vi "AB_RW_Project_RESTfulWebService_Info.vi"(7 "action":T5, 8 "error in (no error)":errorcluster, 10 "RESTfulWebServiceInfo in":T1, 11 "Object In":T6) -> (0 "error out":errorcluster, 2 "RESTfulWebServiceInfo out":T1, 3 "Object Out":T6)   [LabVIEW 2020]
uses:
  <resource>/Framework/Providers/API/ItemRef.ctl
  <vilib>/AppBuilder/RW_Project/AB_RW_Project_PropBag_Action.ctl
  <vilib>/AppBuilder/RW_Project/AB_RW_Project_RESTfulWebService_Data.ctl
  <vilib>/AppBuilder/RW_Project/AB_RW_Project_RESTful_RoutingTemplate.ctl
  <vilib>/AppBuilder/AB_Classes/RESTful/AB_RESTful_RoutingType.ctl
  <vilib>/AppBuilder/AB_Classes/RESTful/AB_RESTful_HTTPMethodType.ctl
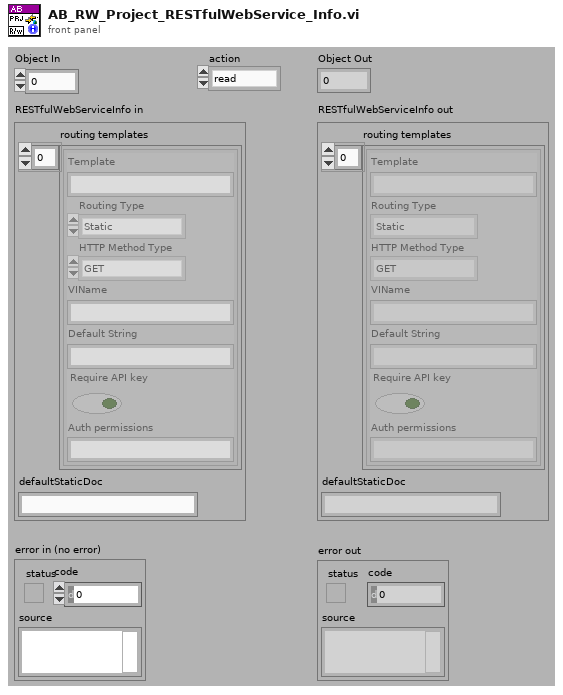
[diagram p1: front panel]
types:
  T1 = typedef "AB_RW_Project_RESTfulWebService_Data.ctl" = cluster{"routing templates":T2[], "defaultStaticDoc":string}
  T2 = typedef "AB_RW_Project_RESTful_RoutingTemplate.ctl" = cluster{"Template":string, "Routing Type":T3, "HTTP Method Type":T4, "VIName":string, "Default String":string, "Require API key":bool, "Auth permissions":string}
  T3 = typedef "AB_RESTful_RoutingType.ctl" = enum32{"Method", "Static"}
  T4 = typedef "AB_RESTful_HTTPMethodType.ctl" = enum32{"GET", "POST", "PUT", "DELETE"}
  T5 = typedef "AB_RW_Project_PropBag_Action.ctl" = enum16{"read", "write", "clear", "readPrevious", "writePrevious", "clearPrevious"}
  T6 = typedef "ItemRef.ctl" = u64
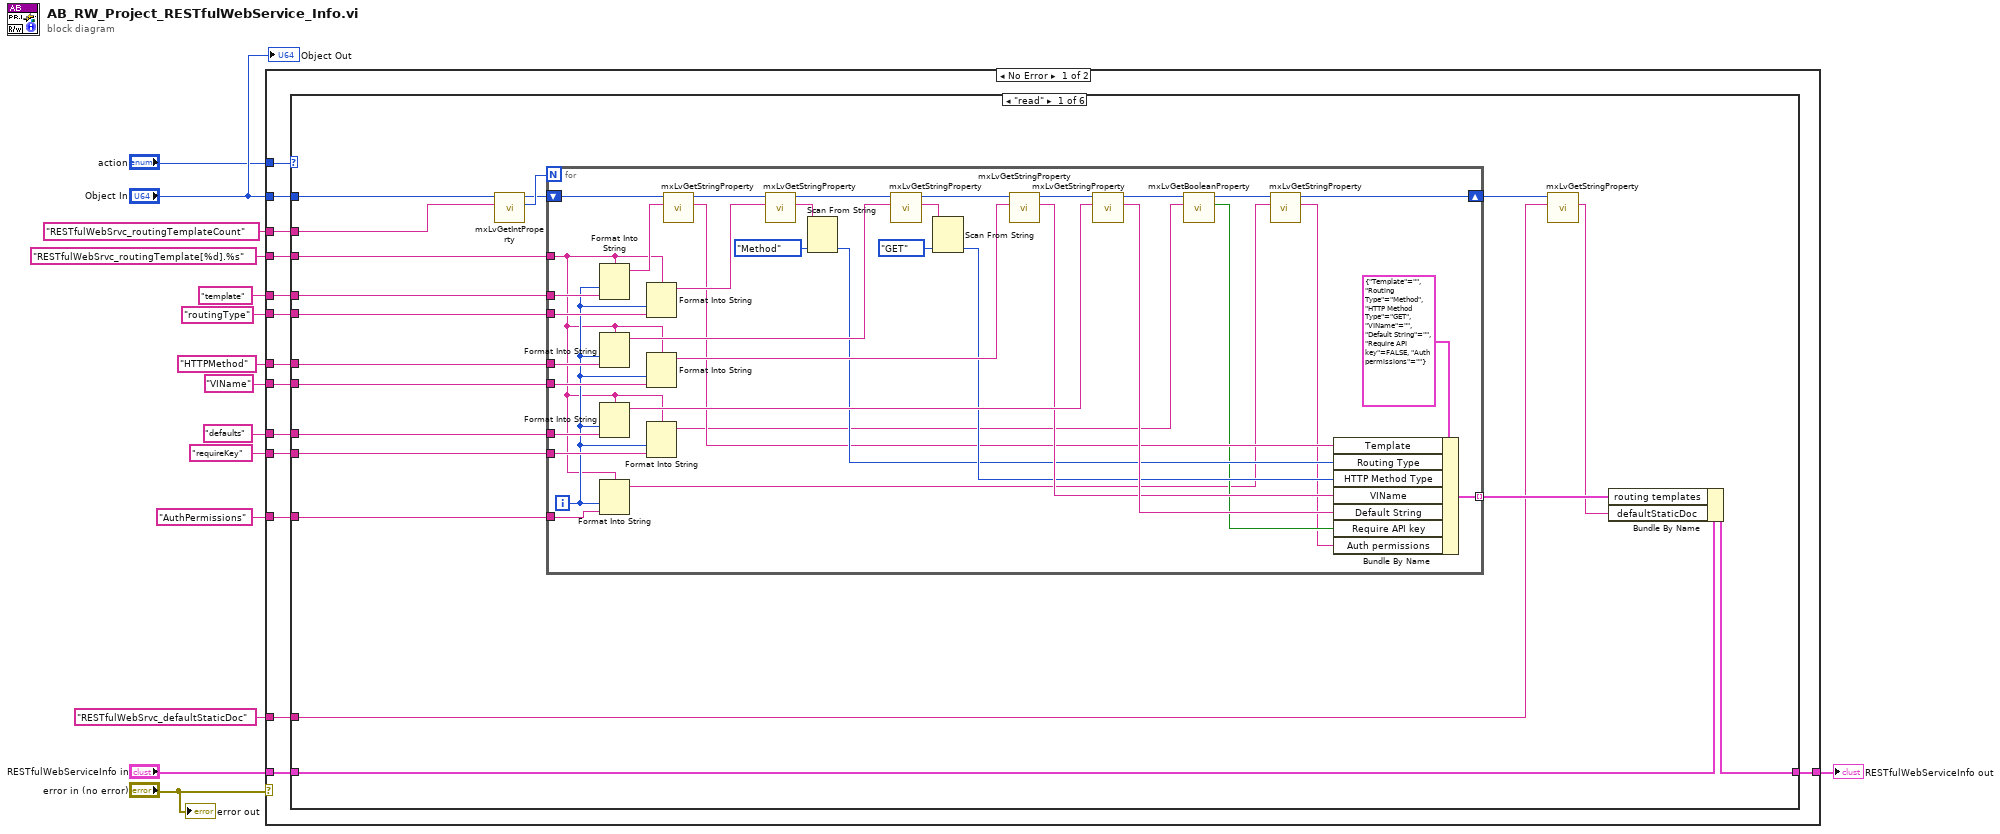
[diagram p0: block diagram]
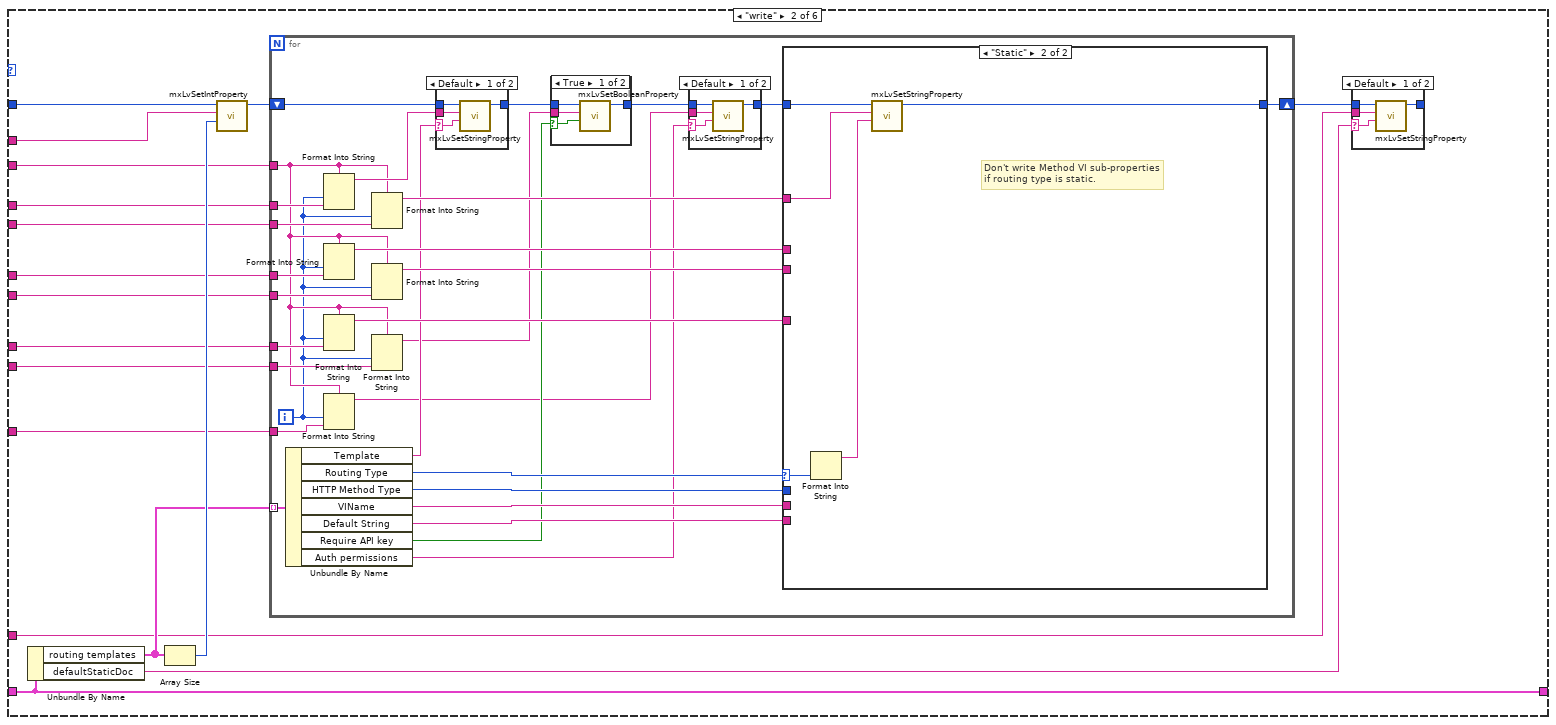
[diagram p2: hidden frame]
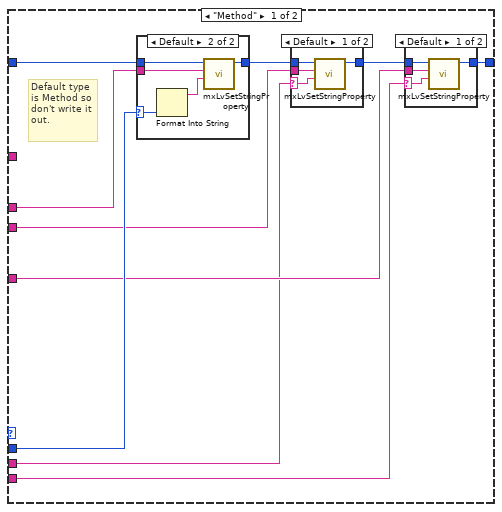
[diagram p6: hidden frame]
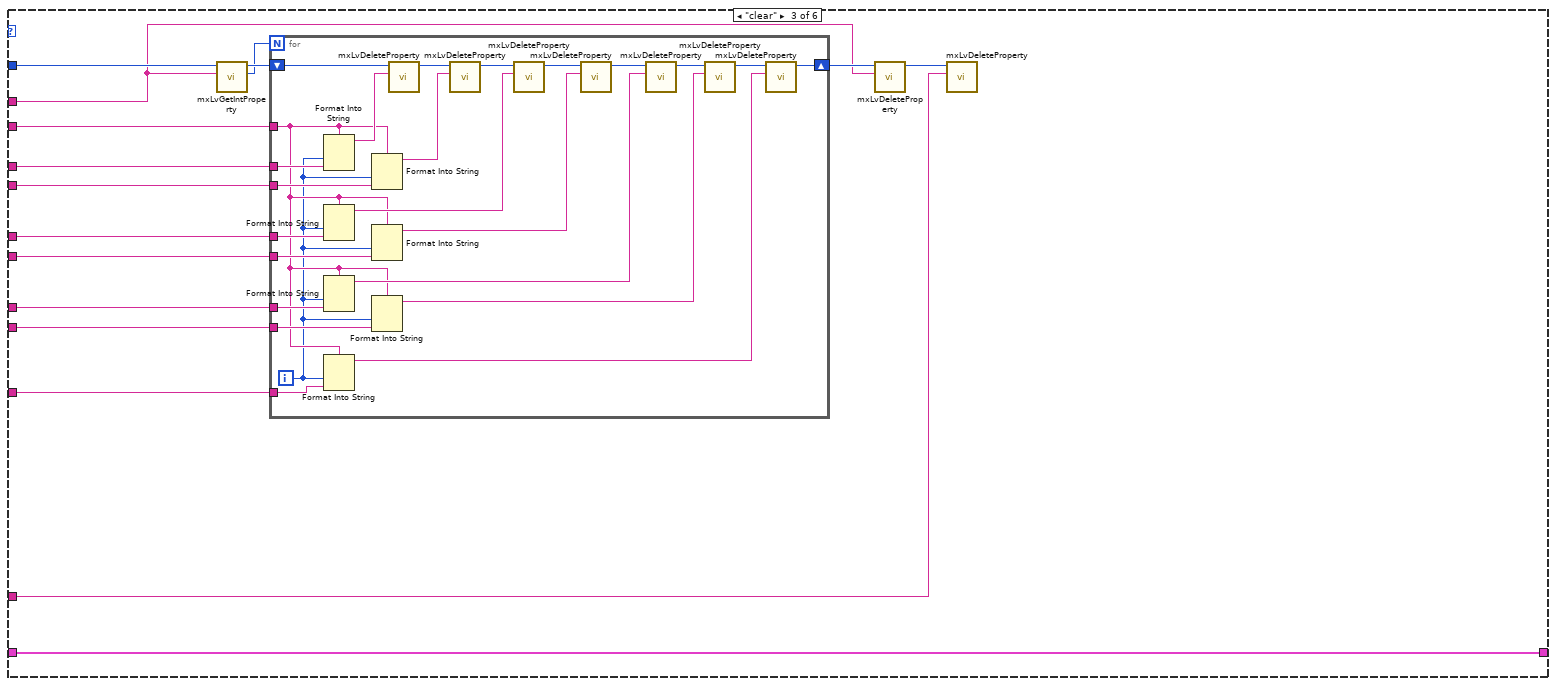
[diagram p11: hidden frame]
diagram:
  n1 = case shown="No Error" "error in (no error)" {
    tunnel: "Object In" -> [w29 _]
    tunnel: [w23 _] -> w8
    tunnel: "RESTfulWebSrvc_routingTemplateCount" ("Tag") -> [w28 _]
    tunnel: "RESTfulWebSrvc_routingTemplate[%d].%s" ("Tag") -> [w27 _]
    tunnel: "template" ("Tag") -> [w26 _]
    tunnel: "RESTfulWebServiceInfo in" -> [w25 _]
    tunnel: "action" -> [w24 _]
    tunnel: "routingType" ("Tag") -> [w22 _]
    tunnel: "HTTPMethod" ("Tag") -> [w21 _]
    tunnel: "VIName" ("Tag") -> [w20 _]
    tunnel: "defaults" ("Tag") -> [w19 _]
    tunnel: "requireKey" ("Tag") -> [w18 _]
    tunnel: "RESTfulWebSrvc_defaultStaticDoc" ("Tag") -> [w17 _]
    tunnel: "AuthPermissions" ("Tag") -> [w16 _]
    frame No Error {
      n2 = case shown="\"read\"" w24 {
        tunnel: w29 -> [w41 w98 w196 _ _ _]
        tunnel: w28 -> [w47 w100 w187 _ _ _]
        tunnel: w27 -> [w45 w96 w194 _ _ _]
        tunnel: w26 -> [w40 w95 w193 _ _ _]
        tunnel: w25 -> [w42 w99 w195 w222 w223 w224]
        tunnel: [w43 w99 w195 w222 w223 w224] -> w23
        tunnel: w22 -> [w39 w94 w192 _ _ _]
        tunnel: w21 -> [w38 w93 w191 _ _ _]
        tunnel: w20 -> [w37 w92 w190 _ _ _]
        tunnel: w19 -> [w36 w91 w189 _ _ _]
        tunnel: w18 -> [w34 w89 w186 _ _ _]
        tunnel: w17 -> [w32 w87 w183 _ _ _]
        tunnel: w16 -> [w30 w85 w182 _ _ _]
        frame "read" {
          n3 = call <resource>:"mxLvGetIntProperty.vi"("Tag"=w47, "Item"=w41) -> ("Value"=w46:i32, "Item"=w44:T6)  [unwired: 1 in, 7 out]
          n4 = for {
            N: w46 -> [_]
            shift-right: [w50] -> w33
            shift-left: w44 -> [w84]
            tunnel: w45 -> [w53]
            tunnel: w40 -> [w81]
            tunnel: w39 -> [w80]
            tunnel: w38 -> [w79]
            tunnel: w37 -> [w78]
            tunnel: w36 -> [w77]
            tunnel: [w60] -> w35 mode=indexing
            tunnel: w34 -> [w57]
            tunnel: w30 -> [w52]
            i -> [w54]
            n5 = Format Into String(format string=w53, w54, w81) -> (resulting string=w76:string)  [unwired: 2 in, 1 out]
            n6 = Format Into String(format string=w53, w54, w79) -> (resulting string=w71:string)  [unwired: 2 in, 1 out]
            n7 = Format Into String(format string=w53, w54, w77) -> (resulting string=w66:string)  [unwired: 2 in, 1 out]
            n8 = Format Into String(format string=w53, w54, w52) -> (resulting string=w48:string)  [unwired: 2 in, 1 out]
            n9 = Format Into String(format string=w53, w54, w80) -> (resulting string=w75:string)  [unwired: 2 in, 1 out]
            n10 = Format Into String(format string=w53, w54, w78) -> (resulting string=w67:string)  [unwired: 2 in, 1 out]
            n11 = Format Into String(format string=w53, w54, w57) -> (resulting string=w56:string)  [unwired: 2 in, 1 out]
            n12 = call <resource>:"mxLvGetStringProperty.vi"("Tag"=w76, "Item"=w84) -> ("Value"=w61:string, "Item"=w83:T6)  [unwired: 1 in, 7 out]
            n13 = call <resource>:"mxLvGetStringProperty.vi"("Tag"=w75, "Item"=w83) -> ("Value"=w82:string, "Item"=w72:T6)  [unwired: 1 in, 7 out]
            n14 = Scan From String(input string=w82, default 1=AB_RESTful_RoutingType."Method" ("Routing Type")) -> (output 1=w62:T3)  [unwired: 3 in, 3 out]
            n15 = call <resource>:"mxLvGetStringProperty.vi"("Tag"=w71, "Item"=w72) -> ("Value"=w73:string, "Item"=w68:T6)  [unwired: 1 in, 7 out]
            n16 = Scan From String(input string=w73, default 1=AB_RESTful_HTTPMethodType."GET" ("HTTP Method Type")) -> (output 1=w63:T4)  [unwired: 3 in, 3 out]
            n17 = call <resource>:"mxLvGetStringProperty.vi"("Tag"=w67, "Item"=w68) -> ("Value"=w64:string, "Item"=w69:T6)  [unwired: 1 in, 7 out]
            n18 = call <resource>:"mxLvGetStringProperty.vi"("Tag"=w66, "Item"=w69) -> ("Value"=w65:string, "Item"=w59:T6)  [unwired: 1 in, 7 out]
            n19 = call <resource>:"mxLvGetBooleanProperty.vi"("Tag"=w56, "Item"=w59) -> ("Value"=w58:bool, "Item"=w51:T6)  [unwired: 1 in, 7 out]
            n20 = call <resource>:"mxLvGetStringProperty.vi"("Tag"=w48, "Item"=w51) -> ("Value"=w49:string, "Item"=w50:T6)  [unwired: 1 in, 7 out]
            n21 = Bundle By Name(cluster=T2 {"Template"="", "Routing Type"=enum."Method", "HTTP Method Type"=enum."GET", "VIName"="", "Default String"="", "Require API key"=FALSE, "Auth permissions"=""} ("RESTful VI routing template"), "Template"=w61, "Routing Type"=w62, "HTTP Method Type"=w63, "VIName"=w64, "Default String"=w65, "Require API key"=w58, "Auth permissions"=w49) -> (w60:T2)
          }
          n22 = call <resource>:"mxLvGetStringProperty.vi"("Tag"=w32, "Item"=w33) -> ("Value"=w31:string)  [unwired: 1 in, 8 out]
          n23 = Bundle By Name(cluster=w42, "routing templates"=w35, "defaultStaticDoc"=w31) -> (w43:T1)
        }
        frame "write" {
          n24 = Unbundle By Name(w99) -> ("routing templates"=w90:T2[], "defaultStaticDoc"=w86:string)
          n25 = Array Size(array=w90) -> (size(s)=w101:i32)
          n26 = call <resource>:"mxLvSetIntProperty.vi"("Value (0)"=w101, "Tag"=w100, "Item"=w98) -> ("Item"=w97:T6)  [unwired: 2 in, 6 out]
          n27 = for {
            shift-right: [w122] -> w88
            shift-left: w97 -> [w119]
            tunnel: w96 -> [w113]
            tunnel: w95 -> [w135]
            tunnel: w94 -> [w134]
            tunnel: w93 -> [w133]
            tunnel: w92 -> [w132]
            tunnel: w91 -> [w131]
            tunnel: w90 -> [w127] mode=indexing
            tunnel: w89 -> [w117]
            tunnel: w85 -> [w111]
            i -> [w112]
            n28 = Unbundle By Name(w127) -> ("Template"=w121:string, "Routing Type"=w118:T3, "HTTP Method Type"=w126:T4, "VIName"=w125:string, "Default String"=w124:string, "Require API key"=w115:bool, "Auth permissions"=w107:string)
            n29 = Format Into String(format string=w113, w112, w135) -> (resulting string=w120:string)  [unwired: 2 in, 1 out]
            n30 = Format Into String(format string=w113, w112, w133) -> (resulting string=w129:string)  [unwired: 2 in, 1 out]
            n31 = Format Into String(format string=w113, w112, w131) -> (resulting string=w123:string)  [unwired: 2 in, 1 out]
            n32 = Format Into String(format string=w113, w112, w111) -> (resulting string=w108:string)  [unwired: 2 in, 1 out]
            n33 = Format Into String(format string=w113, w112, w134) -> (resulting string=w130:string)  [unwired: 2 in, 1 out]
            n34 = Format Into String(format string=w113, w112, w132) -> (resulting string=w128:string)  [unwired: 2 in, 1 out]
            n35 = Format Into String(format string=w113, w112, w117) -> (resulting string=w114:string)  [unwired: 2 in, 1 out]
            n36 = case shown="Default" w121 {
              selector: w121 -> [w177 _]
              tunnel: w119 -> [w180 w181]
              tunnel: w120 -> [w179 _]
              tunnel: [w178 w181] -> w116
              frame Default {
                n37 = call <resource>:"mxLvSetStringProperty.vi"("Value (\"\")"=w177, "Tag"=w179, "Item"=w180) -> ("Item"=w178:T6)  [unwired: 2 in, 6 out]
              }
              frame "" {
              }
            }
            n38 = case shown="True" w115 {
              selector: w115 -> [w143 _]
              tunnel: w116 -> [w144 w145]
              tunnel: w114 -> [w141 _]
              tunnel: [w142 w145] -> w110
              frame True {
                n39 = call <resource>:"mxLvSetBooleanProperty.vi"("Value (F)"=w143, "Tag"=w141, "Item"=w144) -> ("Item"=w142:T6)  [unwired: 2 in, 6 out]
              }
              frame False {
              }
            }
            n40 = case shown="Default" w107 {
              selector: w107 -> [w136 _]
              tunnel: w110 -> [w139 w140]
              tunnel: w108 -> [w138 _]
              tunnel: [w137 w140] -> w109
              frame Default {
                n41 = call <resource>:"mxLvSetStringProperty.vi"("Value (\"\")"=w136, "Tag"=w138, "Item"=w139) -> ("Item"=w137:T6)  [unwired: 2 in, 6 out]
              }
              frame "" {
              }
            }
            n42 = case shown="\"Static\"" w118 {
              selector: w118 -> [_ w172]
              tunnel: w130 -> [_ w173]
              tunnel: w129 -> [w155 _]
              tunnel: w128 -> [w149 _]
              tunnel: w126 -> [w153 _]
              tunnel: w125 -> [w150 _]
              tunnel: w124 -> [w152 _]
              tunnel: w123 -> [w151 _]
              tunnel: [w146 w174] -> w122
              tunnel: w109 -> [w154 w175]
              frame "Method" {
                # "Default type is Method so don't write it out."
                n43 = case shown="Default" w153 {
                  selector: w153 -> [_ w167]
                  tunnel: w155 -> [_ w171]
                  tunnel: [w166 w170] -> w148
                  tunnel: w154 -> [w166 w168]
                  frame "GET" {
                    # "Don't write out default."
                  }
                  frame Default {
                    n44 = Format Into String(w167) -> (resulting string=w169:string)  [unwired: 3 in, 1 out]
                    n45 = call <resource>:"mxLvSetStringProperty.vi"("Value (\"\")"=w169, "Tag"=w171, "Item"=w168) -> ("Item"=w170:T6)  [unwired: 2 in, 6 out]
                  }
                }
                n46 = case shown="Default" w150 {
                  selector: w150 -> [w156 _]
                  tunnel: w148 -> [w159 w160]
                  tunnel: w149 -> [w158 _]
                  tunnel: [w157 w160] -> w147
                  frame Default {
                    n47 = call <resource>:"mxLvSetStringProperty.vi"("Value (\"\")"=w156, "Tag"=w158, "Item"=w159) -> ("Item"=w157:T6)  [unwired: 2 in, 6 out]
                  }
                  frame "" {
                  }
                }
                n48 = case shown="Default" w152 {
                  selector: w152 -> [w161 _]
                  tunnel: w147 -> [w164 w165]
                  tunnel: w151 -> [w163 _]
                  tunnel: [w162 w165] -> w146
                  frame Default {
                    n49 = call <resource>:"mxLvSetStringProperty.vi"("Value (\"\")"=w161, "Tag"=w163, "Item"=w164) -> ("Item"=w162:T6)  [unwired: 2 in, 6 out]
                  }
                  frame "" {
                  }
                }
              }
              frame "Static" {
                # "Don't write Method VI sub-properties if routing type is static."
                n50 = Format Into String(w172) -> (resulting string=w176:string)  [unwired: 3 in, 1 out]
                n51 = call <resource>:"mxLvSetStringProperty.vi"("Value (\"\")"=w176, "Tag"=w173, "Item"=w175) -> ("Item"=w174:T6)  [unwired: 2 in, 6 out]
              }
            }
          }
          n52 = case shown="Default" w86 {
            selector: w86 -> [w102 _]
            tunnel: w88 -> [w105 w106]
            tunnel: w87 -> [w104 _]
            tunnel: [w103 w106] -> _
            frame Default {
              n53 = call <resource>:"mxLvSetStringProperty.vi"("Value (\"\")"=w102, "Tag"=w104, "Item"=w105) -> ("Item"=w103:T6)  [unwired: 2 in, 6 out]
            }
            frame "" {
            }
          }
        }
        frame "clear" {
          n54 = call <resource>:"mxLvGetIntProperty.vi"("Tag"=w187, "Item"=w196) -> ("Value"=w185:i32, "Item"=w197:T6)  [unwired: 1 in, 7 out]
          n55 = for {
            N: w185 -> [_]
            shift-right: [w199] -> w188
            shift-left: w197 -> [w221]
            tunnel: w194 -> [w203]
            tunnel: w193 -> [w219]
            tunnel: w192 -> [w218]
            tunnel: w191 -> [w217]
            tunnel: w190 -> [w216]
            tunnel: w189 -> [w215]
            tunnel: w186 -> [w204]
            tunnel: w182 -> [w201]
            i -> [w202]
            n56 = Format Into String(format string=w203, w202, w219) -> (resulting string=w214:string)  [unwired: 2 in, 1 out]
            n57 = Format Into String(format string=w203, w202, w217) -> (resulting string=w211:string)  [unwired: 2 in, 1 out]
            n58 = Format Into String(format string=w203, w202, w215) -> (resulting string=w207:string)  [unwired: 2 in, 1 out]
            n59 = Format Into String(format string=w203, w202, w201) -> (resulting string=w198:string)  [unwired: 2 in, 1 out]
            n60 = Format Into String(format string=w203, w202, w218) -> (resulting string=w213:string)  [unwired: 2 in, 1 out]
            n61 = Format Into String(format string=w203, w202, w216) -> (resulting string=w208:string)  [unwired: 2 in, 1 out]
            n62 = Format Into String(format string=w203, w202, w204) -> (resulting string=w205:string)  [unwired: 2 in, 1 out]
            n63 = call <resource>:"mxLvDeleteProperty.vi"("Tag"=w214, "Item"=w221) -> ("Item"=w220:T6)  [unwired: 1 in, 8 out]
            n64 = call <resource>:"mxLvDeleteProperty.vi"("Tag"=w213, "Item"=w220) -> ("Item"=w212:T6)  [unwired: 1 in, 8 out]
            n65 = call <resource>:"mxLvDeleteProperty.vi"("Tag"=w211, "Item"=w212) -> ("Item"=w209:T6)  [unwired: 1 in, 8 out]
            n66 = call <resource>:"mxLvDeleteProperty.vi"("Tag"=w208, "Item"=w209) -> ("Item"=w210:T6)  [unwired: 1 in, 8 out]
            n67 = call <resource>:"mxLvDeleteProperty.vi"("Tag"=w207, "Item"=w210) -> ("Item"=w206:T6)  [unwired: 1 in, 8 out]
            n68 = call <resource>:"mxLvDeleteProperty.vi"("Tag"=w205, "Item"=w206) -> ("Item"=w200:T6)  [unwired: 1 in, 8 out]
            n69 = call <resource>:"mxLvDeleteProperty.vi"("Tag"=w198, "Item"=w200) -> ("Item"=w199:T6)  [unwired: 1 in, 8 out]
          }
          n70 = call <resource>:"mxLvDeleteProperty.vi"("Tag"=w187, "Item"=w188) -> ("Item"=w184:T6)  [unwired: 1 in, 8 out]
          n71 = call <resource>:"mxLvDeleteProperty.vi"("Tag"=w183, "Item"=w184) -> ()  [unwired: 1 in, 9 out]
        }
        frame "writePrevious" {
        }
        frame "readPrevious" {
        }
        frame "clearPrevious" {
        }
      }
    }
    frame Error {
    }
  }
  "RESTfulWebServiceInfo out" <- w8
  "Object Out" <- "Object In"
  "error out" <- "error in (no error)"
